vi "Get Motor Power Status_CK.vi"(4 "error in (no error)":errorcluster, 5 "Wait before read (0ms)":u32=5, 6 "Axis (1)":i32=1 min=1 max=3, 7 "VISA resource name":refnum<visa-resource-name>) -> (0 "error out":errorcluster, 2 "Power Status":bool, 3 "VISA resource name out":refnum<visa-resource-name>)   [LabVIEW 2013]
doc: "Get the power status of one axis."
uses:
  <vilib>/Utility/error.llb/whitespace.ctl
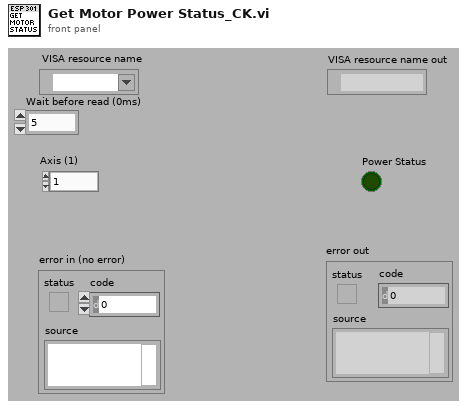
[diagram p1: front panel]
types:
  T1 = typedef "whitespace.ctl" = u16
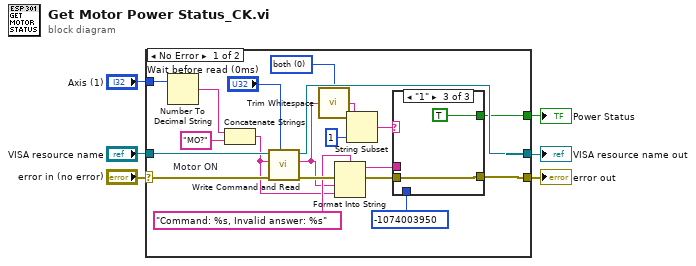
[diagram p0: block diagram]
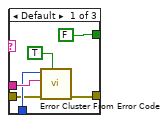
[diagram p2: hidden frame]
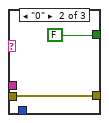
[diagram p3: hidden frame]
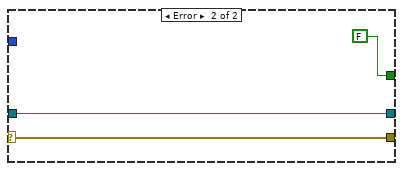
[diagram p4: hidden frame]
diagram:
  n1 = case shown="No Error" "error in (no error)" {
    selector: "error in (no error)" -> [w24 w39]
    tunnel: [w11 w39] -> w6
    tunnel: "VISA resource name" -> [w26 w38]
    tunnel: [w25 w38] -> w5
    tunnel: "Axis (1)" -> [w21 _]
    tunnel: [w15 FALSE ("Motion Done")] -> w1
    frame No Error {
      w9 = T1 0 items=["both", "start of string", "end of string"] ("location (both)")
      w23 = "MO?"  # Motor ON
      n2 = Number To Decimal String(number=w21) -> (decimal integer string=w22:string)  [unwired: 1 in]
      n3 = Concatenate Strings(w22, w23) -> (w13:string)
      n4 = call <instrlib>:"Write Command and Read.vi"("Wait before read (0ms)"="Wait before read (0ms)", "error in (no error)"=w24, "Command"=w13, "VISA resource name"=w26) -> ("error out"=w16:errorcluster, "Returned string"=w8:string, "VISA resource name out"=w25:refnum<visa-resource-name>)  [unwired: 3 in]
      n5 = call <vilib>:"Trim Whitespace.vi"("string"=w8, "location (both)"=w9) -> ("trimmed string"=w7:string)
      n6 = Format Into String(format string="Command: %s, Invalid answer: %s" ("error message (\"\")"), error in=w16, w8, w13) -> (resulting string=w18:string, error out=w12:errorcluster)  [unwired: 1 in]
      n7 = String Subset(string=w7, length (rest)=1 ("longueur (reste)")) -> (substring=w19:string)  [unwired: 1 in]
      n8 = case shown="\"1\"" w19 {
        tunnel: [FALSE ("Motion Done") FALSE ("Motion Done") TRUE ("Motion Done")] -> w15
        tunnel: w18 -> [w30 _ _]
        tunnel: -1074003950 ("error code (0)") -> [w29 _ _]
        tunnel: w12 -> [w28 w33 w35]
        tunnel: [w27 w33 w35] -> w11
        frame Default {
          n9 = call <vilib>:"Error Cluster From Error Code.vi"("show call chain? (False)"=TRUE, "error in (no error)"=w28, "error message (\"\")"=w30, "error code (0)"=w29) -> ("error out"=w27:errorcluster)  [unwired: 5 in]
        }
        frame "0" {
        }
        frame "1" {
        }
      }
    }
    frame Error {
    }
  }
  "error out" <- w6
  "VISA resource name out" <- w5
  "Power Status" <- w1
